vi "set_errorCluster.vi"(0 "error in (no error)":errorcluster, 1 "HGF_Exception":refnum<class "HGF_Exception.lvclass">) -> (2 "dup HGF_Exception":refnum<class "HGF_Exception.lvclass">)   [LabVIEW 2014, in "HGF_BaseClasses.lvlib" / "HGF_Exception.lvclass"]
doc: "This VI overrides the errorCluster attribute."
uses:
  HGF_Exception.lvclass
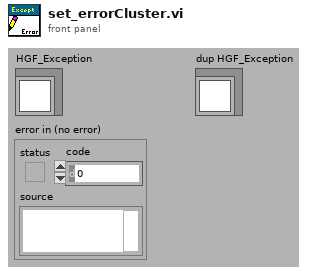
[diagram p1: front panel]
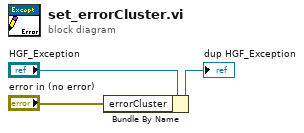
[diagram p0: block diagram]
diagram:
  n1 = Bundle By Name(cluster="HGF_Exception", "errorCluster"="error in (no error)") -> (→"dup HGF_Exception":refnum<class "HGF_Exception.lvclass">)
